vi "Reduce Stock Level and Check.vi"(8 "error in (no error)":errorcluster, 10 "Product Index":i32, 11 "Data Cluster":T1) -> (0 "error out":errorcluster, 2 "Sucessful":bool, 3 "Data Cluster Out":T1)   [LabVIEW 2019, in "Stock.lvlib"]
uses:
  Stock.lvlib
  Module Data--cluster.ctl
  Products.ctl
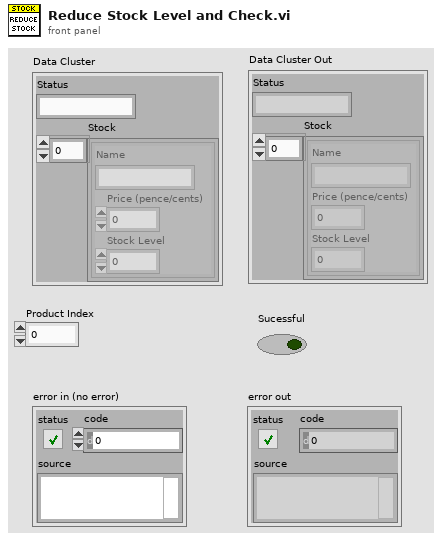
[diagram p1: front panel]
types:
  T1 = typedef "Stock.lvlib/Module Data--cluster.ctl" = cluster{"Status":string, "Stock":T2[]}
  T2 = typedef "Stock.lvlib/Products.ctl" = cluster{"Name":string, "Price (pence/cents)":u32, "Stock Level":u32}
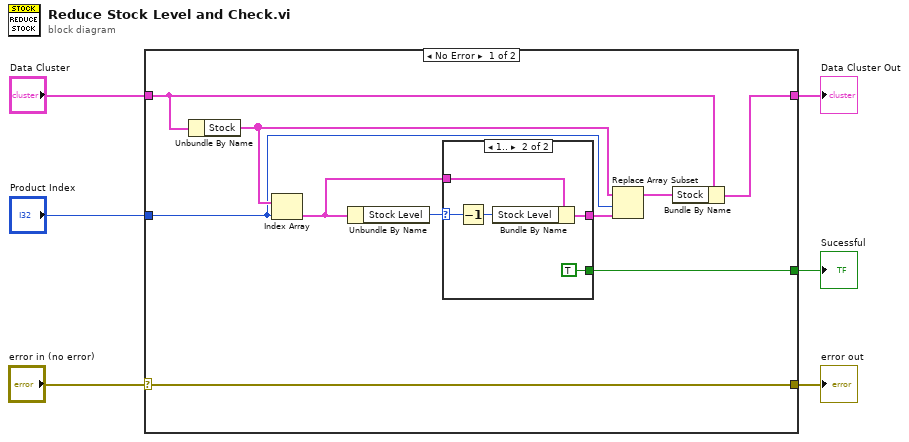
[diagram p0: block diagram]
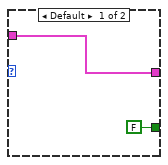
[diagram p2: hidden frame]
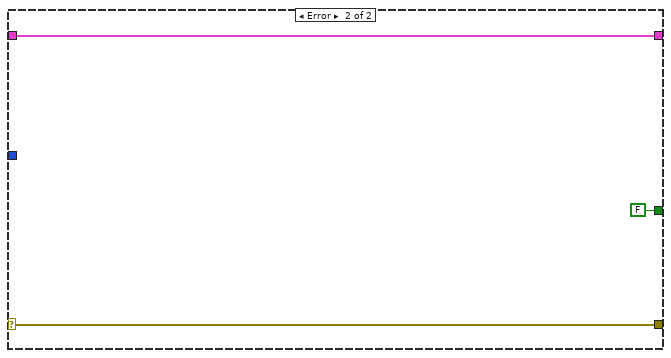
[diagram p3: hidden frame]
diagram:
  n1 = case shown="No Error" "error in (no error)" {
    selector: "error in (no error)" -> [w9 w24]
    tunnel: "Product Index" -> [w7 _]
    tunnel: "Data Cluster" -> [w12 w26]
    tunnel: [w11 w26] -> w4
    tunnel: [w10 FALSE] -> w3
    tunnel: [w9 w24] -> w1
    frame No Error {
      n2 = Unbundle By Name(w12) -> ("Stock"=w15:T2[])
      n3 = Index Array(array=w15, index=w7) -> (element=w16:T2)
      n4 = Unbundle By Name(w16) -> ("Stock Level"=w8:u32)
      n5 = case shown="1.." w8 {
        selector: w8 -> [_ w22]
        tunnel: [FALSE TRUE] -> w10
        tunnel: w16 -> [w17 w23]
        tunnel: [w17 w21] -> w14
        frame Default {
        }
        frame 1.. {
          n6 = Decrement(x=w22) -> (x-1=w19:u32)
          n7 = Bundle By Name(cluster=w23, "Stock Level"=w19) -> (w21:T2)
        }
      }
      n8 = Replace Array Subset(array=w15, new element=w14, index=w7) -> (w13:T2[])
      n9 = Bundle By Name(cluster=w12, "Stock"=w13) -> (w11:T1)
    }
    frame Error {
    }
  }
  "Data Cluster Out" <- w4
  "error out" <- w1
  "Sucessful" <- w3
